vi "FPGA_initialize.vi"   [LabVIEW 2015]
uses:
  <vilib>/rvi/eio/common/nirviEmuTemplateMethod_errors.vi
  <vilib>/eio/EIONode/EIONode.xnode
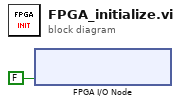
[diagram p0: block diagram]
diagram:
  n1 = xnode "FPGA I/O Node"("Connector0/DIO0"=FALSE) -> ()  [unwired: 1 in, 1 out]
